vi "Display.vi"(8 "error in (no error)":errorcluster, 9 "Line String (This is a comment.)":string="This is a comment.", 10 "Display Page (0: Measurement)":u32(ring) items=["Measurement", "Bin Number", "Bin Count", "List", "Measurement Setup", "Correction Setup", "Limit Table", "List Setup", "System", "Catalog", "SelfTest", "Line String"], 11 "VISA resource name":refnum<visa-resource-name>) -> (0 "error out":errorcluster, 3 "VISA resource name out":refnum<visa-resource-name>)   [LabVIEW 2015, in "Agilent 428X Series.lvlib"]
doc: "The Display VI sets the display page, and enters ASCII characters on the comment line."
uses:
  Agilent 428X Series.lvlib
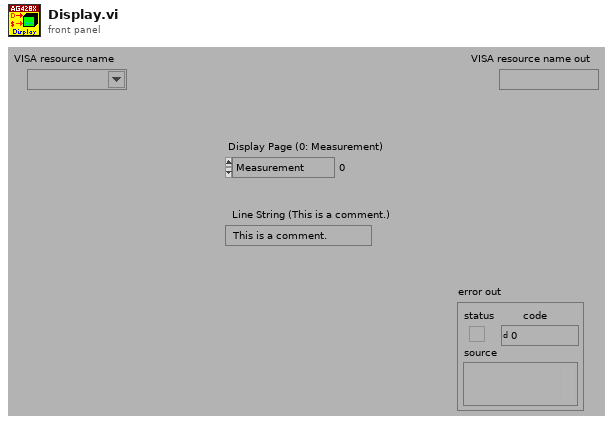
[diagram p1: front panel]
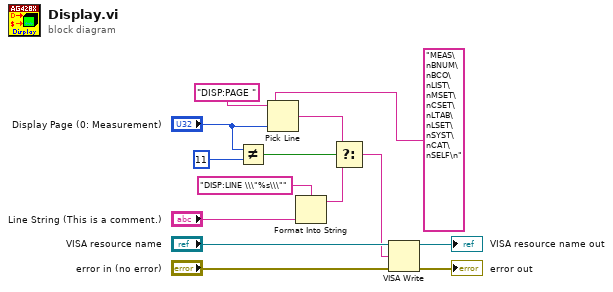
[diagram p0: block diagram]
diagram:
  n1 = Not Equal?(x="Display Page (0: Measurement)", y=u32 11) -> (x != y?=w6:bool)
  n2 = Pick Line(string ("")="DISP:PAGE ", multi-line string="MEAS\nBNUM\nBCO\nLIST\nMSET\nCSET\nLTAB\nLSET\nSYST\nCAT\nSELF\n", line index="Display Page (0: Measurement)") -> (output string=w5:string)
  n3 = Format Into String(format string="DISP:LINE \\\"%s\\\"", "Line String (This is a comment.)") -> (resulting string=w2:string)  [unwired: 2 in, 1 out]
  n4 = Select(t=w5, s=w6, f=w2) -> (s? t:f=w1:string)
  n5 = VISA Write(VISA resource name="VISA resource name", write buffer=w1, error in (no error)="error in (no error)") -> (VISA resource name out=→"VISA resource name out":refnum<visa-resource-name>, error out=→"error out":errorcluster)  [unwired: 1 out]
